vi "No._to_Gulton_string_mrw.vi"(2 "PARAMETER":dbl format="%.2f", 3 "INPUT VALUE":dbl format="%.2f") -> (1 "OUTPUT STRING":string)   [LabVIEW 2010]
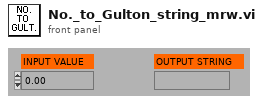
[diagram p1: front panel]
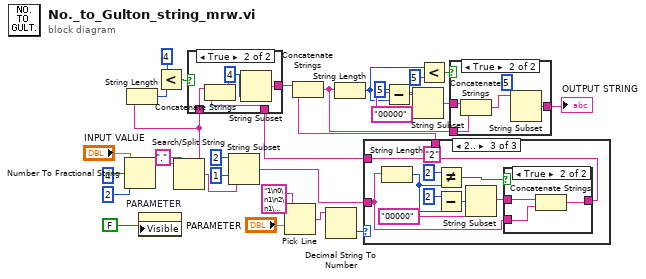
[diagram p0: block diagram]
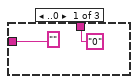
[diagram p2: hidden frame]
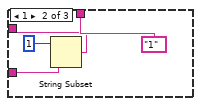
[diagram p3: hidden frame]
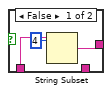
[diagram p6: hidden frame]
diagram:
  n1 = Number To Fractional String(number="INPUT VALUE", width (-)=4, precision (6)=2) -> (F-format string=w6:string)  [unwired: 1 in]
  n2 = property on="PARAMETER" class="DigNum (strict)"("Visible"=FALSE) -> ()  [unwired: 2 in, 2 out]
  n3 = Search/Split String(string=w6, search string/char (-)=".") -> (substring before match=w8:string, match + rest of string=w12:string)  [unwired: 1 in, 1 out]
  n4 = String Length(string=w8) -> (length=w28:i32)
  n5 = Less?(x=w28, y=4) -> (x < y?=w27:bool)
  n6 = String Subset(string=w12, offset (0)=1, length (rest)=2) -> (substring=w5:string)
  n7 = Pick Line(multi-line string="1\n0\n1\n2\n1\n1\n2\n1\n1\n1\n1\n1\n1\n1", line index="PARAMETER") -> (output string=w2:string)  [unwired: 1 in]
  n8 = Decimal String To Number(string=w2) -> (number=w1:i32)  [unwired: 2 in, 1 out]
  n9 = case shown="2.." w1 {
    tunnel: ["" w33 w44] -> w11
    tunnel: w5 -> [_ w34 w43]
    tunnel: ["0" "1" "2"] -> w13
    frame ..0 {
    }
    frame 1 {
      n10 = String Subset(string=w34, length (rest)=1) -> (substring=w33:string)  [unwired: 1 in]
    }
    frame 2.. {
      n11 = String Length(string=w43) -> (length=w38:i32)
      n12 = Not Equal?(x=2, y=w38) -> (x != y?=w41:bool)
      n13 = Subtract(x=2, y=w38) -> (x-y=w46:i32)
      n14 = String Subset(string="00000", length (rest)=w46) -> (substring=w40:string)  [unwired: 1 in]
      n15 = case shown="True" w41 {
        tunnel: w40 -> [_ w49]
        tunnel: [w47 w48] -> w44
        tunnel: w43 -> [w47 w50]
        frame False {
        }
        frame True {
          n16 = Concatenate Strings(w50, w49) -> (w48:string)
        }
      }
    }
  }
  n17 = case shown="True" w27 {
    tunnel: w11 -> [_ w54]
    tunnel: w8 -> [w52 w58]
    tunnel: [w51 w55] -> w10
    frame False {
      n18 = String Subset(string=w52, length (rest)=4) -> (substring=w51:string)  [unwired: 1 in]
    }
    frame True {
      n19 = Concatenate Strings(w58, w54) -> (w56:string)
      n20 = String Subset(string=w56, length (rest)=4) -> (substring=w55:string)  [unwired: 1 in]
    }
  }
  n21 = Concatenate Strings(w10, w13) -> (w18:string)
  n22 = String Length(string=w18) -> (length=w9:i32)
  n23 = Subtract(x=5, y=w9) -> (x-y=w19:i32)
  n24 = String Subset(string="00000", length (rest)=w19) -> (substring=w7:string)  [unwired: 1 in]
  n25 = Less?(x=w9, y=5) -> (x < y?=w17:bool)
  n26 = case shown="True" w17 {
    tunnel: [w59 w63] -> w20
    tunnel: w18 -> [w59 w62]
    tunnel: w7 -> [_ w61]
    frame False {
    }
    frame True {
      n27 = Concatenate Strings(w61, w62) -> (w60:string)
      n28 = String Subset(string=w60, length (rest)=5) -> (substring=w63:string)  [unwired: 1 in]
    }
  }
  "OUTPUT STRING" <- w20
